vi "3.饼状图计数.vi"(8 "error in":errorcluster, 10 "Pass(T) Fail(F)":bool, 11 "Module ID":i32=-1) -> (0 "error out":errorcluster, 3 "Module ID out":i32=-1)   [LabVIEW 2020, in "PichartInterface.lvlib"]
uses:
  PichartInterface.lvlib
  <vilib>/DD/DDToolsVIPM/PieChartInterface/PieChart.lvlibp
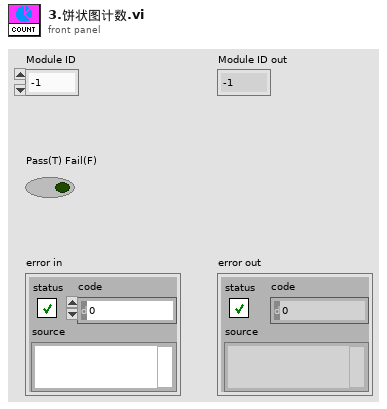
[diagram p1: front panel]
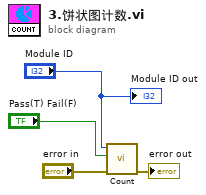
[diagram p0: block diagram]
diagram:
  n1 = call <vilib>:"Count.vi"("error in"="error in", "Pass(T) Fail(F)"="Pass(T) Fail(F)", "Module ID"="Module ID") -> ("error out"=→"error out":errorcluster)  [unwired: 8 in]
  "Module ID out" <- "Module ID"
